vi "VE.vi"(8 "error in (no error)":errorcluster, 11 "Agilis in":T1) -> (0 "error out":errorcluster, 2 "Firmware Version":string, 3 "Agilis out":T1)   [LabVIEW 2016, in "Drivers.lvlib" / "Agilis.lvlib"]
doc: "Returns the firmware version of the controller."
uses:
  Agilis.lvlib
  AgilisCmdLib Refnum.ctl
  Z:/TraceGrabber/Drivers/Agilis/AgilisCmdLib.dll
  AgilisCmdLib.dll
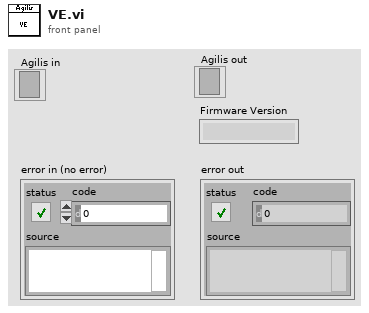
[diagram p1: front panel]
types:
  T1 = typedef "Drivers.lvlib/Agilis.lvlib/AgilisCmdLib Refnum.ctl" = refnum<k24>
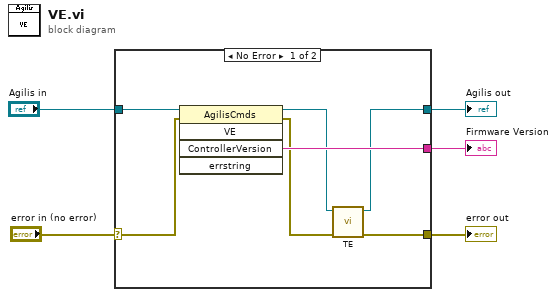
[diagram p0: block diagram]
diagram:
  n1 = case shown="No Error" "error in (no error)" {
    selector: "error in (no error)" -> [w11 w14]
    tunnel: "Agilis in" -> [w12 w13]
    tunnel: [w6 w13] -> w3
    tunnel: [w8 w14] -> w2
    tunnel: [w10 _] -> w1
    frame No Error {
      n2 = invoke class="AgilisCmds" method="VE"(reference=w12, error in=w11) -> (reference out=w7:T1, error out=w9:errorcluster, "ControllerVersion"=w10:string)  [unwired: 3 in, 2 out]
      n3 = call "TE.vi"("error in (no error)"=w9, "Agilis in"=w7) -> ("error out"=w8:errorcluster, "Agilis out"=w6:T1)  [unwired: 8 in]
    }
    frame Error {
    }
  }
  "Agilis out" <- w3
  "error out" <- w2
  "Firmware Version" <- w1
